vi "SW_Type_1c_correction.vi"(1 "variable n":bool, 2 "wire diameter (mu.m)":dbl=5.0, 3 "calib consts. t":dbl[](array[numeric]), 4 "calib consts. t1":dbl[](array[numeric])) -> (0 "Corrected calib consts. t":dbl[](array[numeric]))   [LabVIEW 2011]
panel:
  # "Type 1c: Correct intermediate \"calibration\" constants at tk, but with conditions at ti,  to conditions at tk"
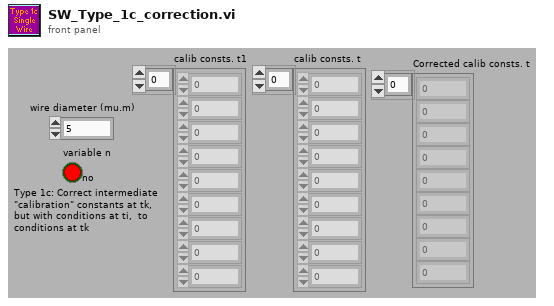
[diagram p1: front panel]
types:
  T1 = cluster{"calib consts. t1[0]":dbl, "calib consts. t1[1]":dbl, "calib consts. t1[2]":dbl, "calib consts. t1[3]":dbl, "calib consts. t1[4]":dbl, "calib consts. t1[5]":dbl, "calib consts. t1[6]":dbl, "calib consts. t1[7]":dbl}
  T2 = cluster{"calib consts. t[0]":dbl, "calib consts. t[1]":dbl, "calib consts. t[2]":dbl, "calib consts. t[3]":dbl, "calib consts. t[4]":dbl, "calib consts. t[5]":dbl, "calib consts. t[6]":dbl, "calib consts. t[7]":dbl}
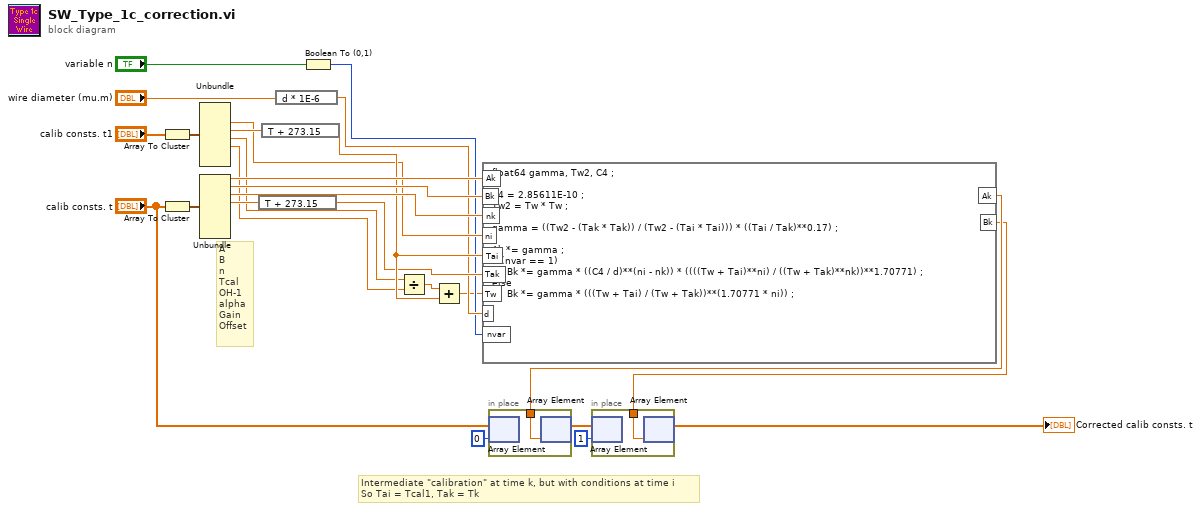
[diagram p0: block diagram]
diagram:
  # "Intermediate \"calibration\" at time k, but with conditions at time i\nSo Tai = Tcal1, Tak = Tk"
  # "A\nB\nn\nTcal\nOH-1\nalpha\nGain\nOffset"
  n1 = Array To Cluster(array="calib consts. t1") -> (cluster=w17:T1)
  n2 = Array To Cluster(array="calib consts. t") -> (cluster=w26:T2)
  n3 = Unbundle(w17) -> ("calib consts. t1[2]"=w13:dbl, "calib consts. t1[3]"=w15:dbl, "calib consts. t1[4]"=w14:dbl, "calib consts. t1[5]"=w1:dbl)  [unwired: 4 out]
  n4 = Unbundle(w26) -> ("calib consts. t[0]"=w25:dbl, "calib consts. t[1]"=w24:dbl, "calib consts. t[2]"=w23:dbl, "calib consts. t[3]"=w20:dbl)  [unwired: 4 out]
  n5 = expression code="T + 273.15"(w20) -> (w19:dbl)
  n6 = expression code="T + 273.15"(w15) -> (w21:dbl)
  n7 = expression code="d * 1E-6"("wire diameter (mu.m)") -> (w11:dbl)
  n8 = Boolean To (0,1)(Boolean="variable n") -> (0, 1=w9:i16)
  n9 = Divide(x=w14, y=w1) -> (x/y=w8:dbl)
  n10 = Add(x=w8, y=w21) -> (x+y=w7:dbl)
  n11 = formula code="float64 gamma, Tw2, C4 ;\n\nC4 = 2.85611E-10 ;\nTw2 = Tw * Tw ;\n\ngamma = ((Tw2 - (Tak * Tak)) / (Tw2 - (Tai * Tai))) * ((Tai / Tak)**0.17) ;\n\nAk *= gamma ;\nif (nvar == 1)\n     Bk *= gamma * ((C4 / d)**(ni - nk)) * ((((Tw + Tai)**ni) / ((Tw + Tak)**nk))**1.70771) ;\nelse\n     Bk *= gamma * (((Tw + Tai) / (Tw + Tak))**(1.70771 * ni)) ;"("Ak"=w25, "Bk"=w24, "nk"=w23, "Tai"=w21, "Tak"=w19, "Tw"=w7, "ni"=w13, "d"=w11, "nvar"=w9) -> ("Ak"=w5:dbl, "Bk"=w4:dbl)
  n12 = in-place {
    in-place-border: w5 -> [w27]
    n13 = in-place-array #1("calib consts. t", 0) -> ()  [unwired: 1 out]
    n14 = in-place-array #1(w27) -> (w2:dbl[])  [unwired: 1 out]
  }
  n15 = in-place {
    in-place-border: w4 -> [w28]
    n16 = in-place-array #2(w2, 1) -> ()  [unwired: 1 out]
    n17 = in-place-array #2(w28) -> (→"Corrected calib consts. t":dbl[])  [unwired: 1 out]
  }
